vi "test_Add ByteCount Response_UseChannel.vi"(8 "error in (no error)":errorcluster, 11 "TestCase in":refnum<class "Instrument Addon Scripting API Messages Unit Tests.lvclass">) -> (0 "error out":errorcluster, 3 "TestCase out":refnum<class "Instrument Addon Scripting API Messages Unit Tests.lvclass">)   [LabVIEW 2018, in "Instrument Addon Scripting API Messages Unit Tests.lvclass"]
uses:
  Instrument Addon Scripting API Messages Unit Tests.lvclass
  APIs/Scripting API/TypeDefs/ByteCount Response Settings.ctl
  APIs/Scripting API/TypeDefs/Linked Channel.ctl
  <vilib>/NI Veristand/Custom Device API/Custom Device Item Ref.ctl
  Addon/Addon Shared/Types/Response Parameters.ctl
  Addon/Addon Shared/Types/Linked Channel Cluster.ctl
  Addon/Addon Shared/Types/Response Wait Type.ctl
  Addon/Addon Shared/Types/FG Control.ctl
  Addon/Addon Shared/SubVIs/Constants.vi
  <vilib>/NI/NI VeriStand Advanced SysDef API/_SubVIs/SysDef.Search.GUID.vi
  <vilib>/NI Veristand/Custom Device API/NI VeriStand - Get Item Property.vi
  <vilib>/NI Veristand/Custom Device API/Get Item Property (String).vi
  <vilib>/NI Veristand/Custom Device API/Get Item Property (String Array).vi
  <vilib>/NI Veristand/Custom Device API/Get Item Property (Double).vi
  <vilib>/NI Veristand/Custom Device API/Get Item Property (U32).vi
  <vilib>/NI Veristand/Custom Device API/Get Item Property (Boolean).vi
  <vilib>/NI Veristand/Custom Device API/NI VeriStand - Set Item Property.vi
  <vilib>/NI Veristand/Custom Device API/Set Item Property (String).vi
  <vilib>/NI Veristand/Custom Device API/Set Item Property (String Array).vi
  <vilib>/NI Veristand/Custom Device API/Set Item Property (Double).vi
  <vilib>/NI Veristand/Custom Device API/Set Item Property (U32).vi
  <vilib>/NI Veristand/Custom Device API/Set Item Property (Boolean).vi
  APIs/Scripting API/Messages/Add Response - Byte Count.vi
  <vilib>/addons/_JKI Toolkits/VI Tester/TestCase.llb/TestCase.lvclass
  Instrument Addon Scripting API Test Assets/Instrument Addon Scripting API Test Assets.lvclass
  APIs/Scripting API/Instrument Addon Scripting API.lvlib
  <vilib>/NI Veristand/Custom Device API/Custom Device API.lvlib
  Addon/Addon Shared/Instrument Addon Shared.lvlib
  <vilib>/NI/NI VeriStand Advanced SysDef API/SysDef API/Advanced System Definition.lvlib
  C:/Program Files (x86)/National Instruments/LabVIEW 2018/vi.lib/addons/_JKI Toolkits/VI Tester/TestCase.llb/TestCase.lvclass
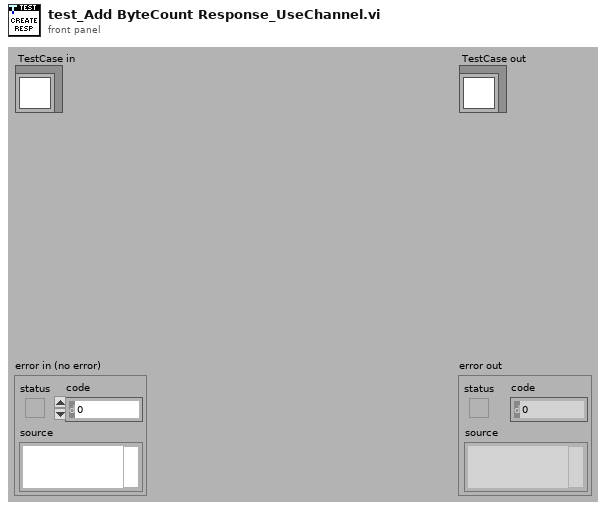
[diagram p1: front panel]
types:
  T1 = typedef "Instrument Addon Shared.lvlib/FG Control.ctl" = enum16{"Get", "Set"}
  T2 = typedef "Custom Device API.lvlib/Custom Device Item Ref.ctl" = u64
  T3 = typedef "Instrument Addon Scripting API.lvlib/Linked Channel.ctl" = cluster{"Variable Name":string, "Channel Refnum":T2}
  T4 = typedef "Instrument Addon Scripting API.lvlib/ByteCount Response Settings.ctl" = cluster{"Response Format":string, "Linked Channels":T3[], "Byte Count":i32, "Use Byte Count channel":bool, "Channel Refnum":T2}
  T5 = typedef "Instrument Addon Shared.lvlib/Response Parameters.ctl" = cluster{"Response":string, "Linked Channels":T6[], "Type Value":dbl, "Wait Type":T7, "Use Channel":bool, "Channel Path":string}
  T6 = typedef "Instrument Addon Shared.lvlib/Linked Channel Cluster.ctl" = cluster{"Variable Name":string, "GUID":string}
  T7 = typedef "Instrument Addon Shared.lvlib/Response Wait Type.ctl" = enum16{"Byte Count", "Wait sec"}
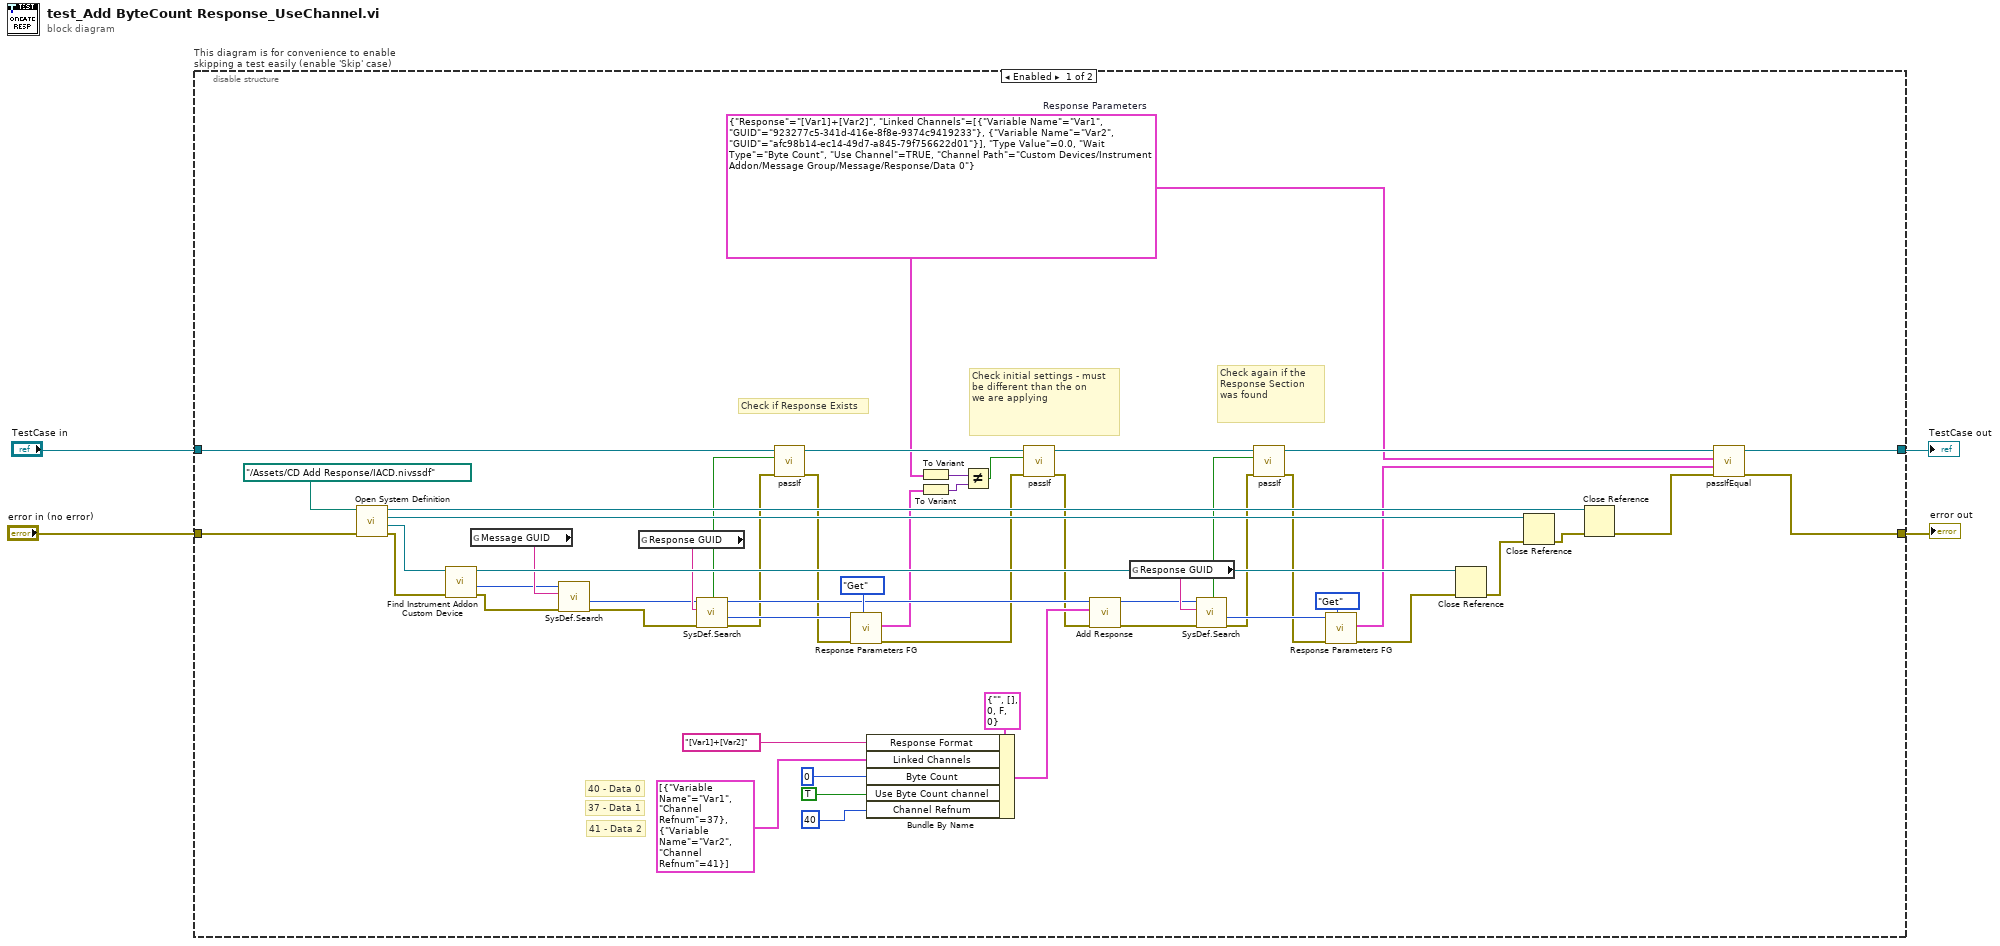
[diagram p0: block diagram]
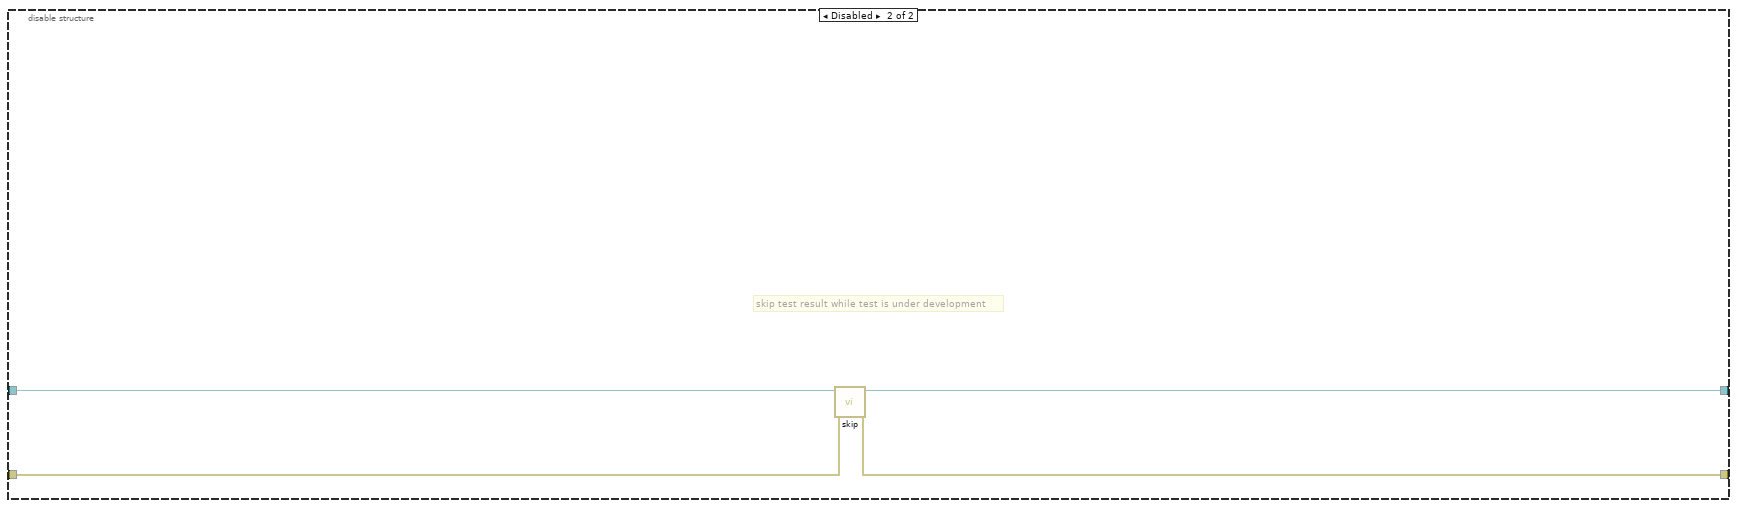
[diagram p2: hidden frame]
diagram:
  n1 = disable-structure "This diagram is for convenience to enable skipping a test easily (enable 'Skip' case)" shown="Enabled" {
    disable-tunnel: "TestCase in" -> [w21 w60]
    disable-tunnel: [w33 w58] -> w1
    disable-tunnel: [w32 w59] -> w3
    disable-tunnel: "error in (no error)" -> [w55 w57]
    frame Enabled {
      w5 = T5 {"Response"="[Var1]+[Var2]", "Linked Channels"=[{"Variable Name"="Var1", "GUID"="923277c5-341d-416e-8f8e-9374c9419233"}, {"Variable Name"="Var2", "GUID"="afc98b14-ec14-49d7-a845-79f756622d01"}], "Type Value"=0.0, "Wait Type"=enum."Byte Count", "Use Channel"=TRUE, "Channel Path"="Custom Devices/Instrument Addon/Message Group/Message/Response/Data 0"}  # Response Parameters
      # "Check again if the Response Section was found"
      # "Check initial settings - must be different than the on\nwe are applying"
      # "Check if Response Exists"
      # "41 - Data 2"
      # "40 - Data 0"
      # "37 - Data 1"
      n2 = call "Open System Definition.vi"("error in (no error)"=w55, "System Definition File"=path "../Assets/CD Add Response/IACD.nivssdf" ("SDF file")) -> ("error out"=w53:errorcluster, "Target Refnum"=w52:refnum<k24>, "Root Refnum"=w51:refnum<k24>, "System Definition Refnum"=w36:refnum<k24>)  [unwired: 6 in]
      n3 = call "Find Instrument Addon Custom Device.vi"("error in"=w53, "target in"=w52) -> ("error out"=w10:errorcluster, "NodeID"=w7:u64, "target out"=w50:refnum<k24>)  [unwired: 7 in]
      n4 = global read "Constants.vi" "Message GUID"() -> (w8:string)
      n5 = call-poly <vilib>:"SysDef.Search.vi"("error in (no error)"=w10, "GUID"=w8, "nodeID"=w7) -> ("error out"=w9:errorcluster, "Value out"=w6:u64)  [unwired: 5 in, 2 out]
      n6 = global read "Constants.vi" "Response GUID"() -> (w29:string)
      n7 = call-poly <vilib>:"SysDef.Search.vi"("error in (no error)"=w9, "GUID"=w29, "nodeID"=w6) -> ("error out"=w19:errorcluster, "Value out"=w30:u64, "nodeID out"=w28:u64, "Found?"=w20:bool)  [unwired: 5 in]
      n8 = call-dynamic "passIf.vi"("error in (no error)"=w19, "pass"=w20, "TestCase in"=w21) -> ("error out"=w18:errorcluster, "TestCase out"=w17:refnum<class "Instrument Addon Scripting API Messages Unit Tests.lvclass">)  [unwired: 7 in]
      n9 = call "Response Parameters FG.vi"("Action"=FG_Control."Get", "error in (no error)"=w18, "Item Ref in"=w30) -> ("error out"=w16:errorcluster, "Response Parameters"=w27:T5)  [unwired: 6 in, 1 out]
      n10 = Bundle By Name(cluster=T4 {"Response Format"="", "Linked Channels"=[], "Byte Count"=0, "Use Byte Count channel"=FALSE, "Channel Refnum"=0} ("Settings"), "Response Format"="[Var1]+[Var2]", "Linked Channels"=T3[] [{"Variable Name"="Var1", "Channel Refnum"=37}, {"Variable Name"="Var2", "Channel Refnum"=41}], "Byte Count"=0, "Use Byte Count channel"=TRUE, "Channel Refnum"=T2 40) -> (w43:T4)
      n11 = To Variant(anything=w5) -> (Variant=w26:variant)
      n12 = To Variant(anything=w27) -> (Variant=w25:variant)
      n13 = Not Equal?(x=w26, y=w25) -> (x != y?=w24:bool)
      n14 = call-dynamic "passIf.vi"("error in (no error)"=w16, "pass"=w24, "TestCase in"=w17) -> ("error out"=w23:errorcluster, "TestCase out"=w15:refnum<class "Instrument Addon Scripting API Messages Unit Tests.lvclass">)  [unwired: 7 in]
      n15 = call-poly "Add Response.vi"("error in (no error)"=w23, "Settings"=w43, "Message in"=w28) -> ("error out"=w39:errorcluster, "Message out"=w38:T2)  [unwired: 7 in]
      n16 = global read "Constants.vi" "Response GUID"() -> (w40:string)
      n17 = call-poly <vilib>:"SysDef.Search.vi"("error in (no error)"=w39, "GUID"=w40, "nodeID"=w38) -> ("error out"=w14:errorcluster, "Value out"=w37:u64, "Found?"=w13:bool)  [unwired: 5 in, 1 out]
      n18 = call-dynamic "passIf.vi"("error in (no error)"=w14, "pass"=w13, "TestCase in"=w15) -> ("error out"=w12:errorcluster, "TestCase out"=w11:refnum<class "Instrument Addon Scripting API Messages Unit Tests.lvclass">)  [unwired: 7 in]
      n19 = call "Response Parameters FG.vi"("Action"=FG_Control."Get", "error in (no error)"=w12, "Item Ref in"=w37) -> ("error out"=w41:errorcluster, "Response Parameters"=w22:T5)  [unwired: 6 in, 1 out]
      n20 = Close Reference(reference=w50, error in (no error)=w41) -> (error out=w54:errorcluster)
      n21 = Close Reference(reference=w51, error in (no error)=w54) -> (error out=w35:errorcluster)
      n22 = Close Reference(reference=w36, error in (no error)=w35) -> (error out=w34:errorcluster)
      n23 = call-dynamic "passIfEqual.vi"("error in (no error)"=w34, "y"=w22, "x"=w5, "TestCase in"=w11) -> ("error out"=w32:errorcluster, "TestCase out"=w33:refnum<class "Instrument Addon Scripting API Messages Unit Tests.lvclass">)  [unwired: 6 in]
    }
    frame Disabled {
      # "skip test result while test is under development"
      n24 = call <vilib>:"skip.vi"("error in (no error)"=w57, "TestCase in"=w60) -> ("error out"=w59:errorcluster, "TestCase out"=w58:refnum<class "Instrument Addon Scripting API Messages Unit Tests.lvclass">)  [unwired: 8 in]
    }
  }
  "error out" <- w3
  "TestCase out" <- w1
